vi "writeU32.vi"(8 "error in (no error)":errorcluster, 10 "Input":u32, 11 "M1M3SAL in":refnum<class "M1M3SAL.lvclass">) -> (0 "error out":errorcluster, 3 "M1M3SAL out":refnum<class "M1M3SAL.lvclass">)   [LabVIEW 2016, in "M1M3SupportCommunicator.lvlib" / "M1M3SAL.lvclass"]
uses:
  M1M3SAL.lvclass
  M1M3SAL.lvclass/M1M3SAL.ctl
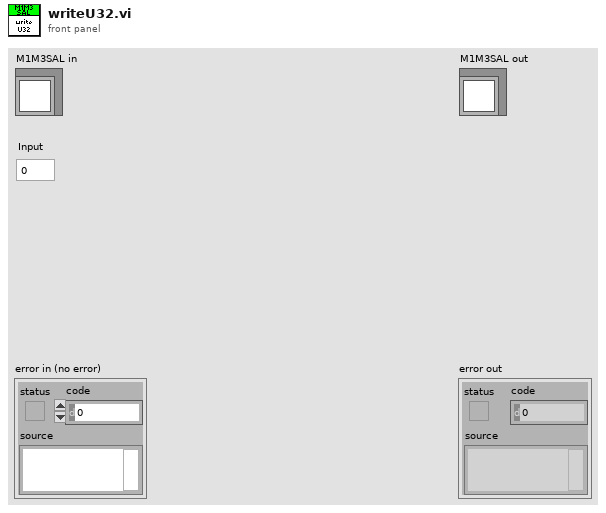
[diagram p1: front panel]
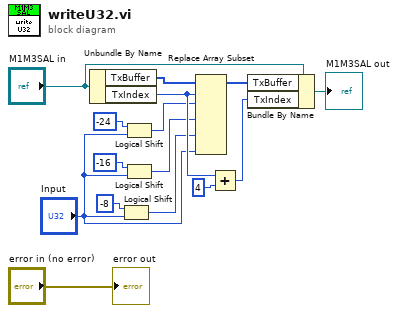
[diagram p0: block diagram]
diagram:
  n1 = Unbundle By Name("M1M3SAL in") -> ("TxBuffer"=w13:u8[], "TxIndex"=w12:i32)
  n2 = Logical Shift(y=i16 -8, x="Input") -> (x << y=w2:u32)
  n3 = Logical Shift(y=i16 -24, x="Input") -> (x << y=w4:u32)
  n4 = Logical Shift(y=i16 -16, x="Input") -> (x << y=w3:u32)
  n5 = Replace Array Subset(array=w13, new element #1=w4, index #1=w12, new element #2=w3, new element #3=w2, new element #4="Input") -> (w9:u8[])  [unwired: 3 in]
  n6 = Add(x=w12, y=4) -> (x+y=w10:i32)
  n7 = Bundle By Name(cluster="M1M3SAL in", "TxBuffer"=w9, "TxIndex"=w10) -> (→"M1M3SAL out":refnum<class "M1M3SAL.lvclass">)
  "error out" <- "error in (no error)"
